vi "Add Device.vi"(8 "error in (no error)":errorcluster, 9 "J1939 Monitor Settings":T2 {"Name" format="%.0x"}, 10 "Name":string, 11 "NodeID":u64) -> (0 "error out":errorcluster, 2 "Device Ref out":T1 format="%.0x")   [LabVIEW 2023, in "J1939 System Definition API Support.lvlib"]
uses:
  J1939 System Definition API Support.lvlib
  Addon/Addon Shared/Types/Monitor Settings.ctl
  <vilib>/NI VeriStand/Custom Device API/Custom Device Item Ref.ctl
  Addon/Addon Shared/SubVIs/Constants.vi
  <vilib>/NI/NI VeriStand Advanced SysDef API/_SubVIs/SysDef.Search.GUID.vi
  Addon/Addon Shared/J1939 Addon Shared.lvlib
  <vilib>/NI/NI VeriStand Advanced SysDef API/SysDef API/Advanced System Definition.lvlib
  <vilib>/NI VeriStand/Custom Device API/Custom Device API.lvlib
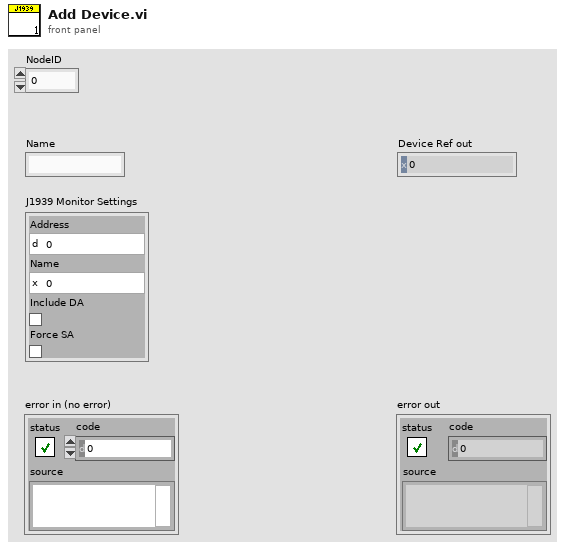
[diagram p1: front panel]
types:
  T1 = typedef "Custom Device API.lvlib/Custom Device Item Ref.ctl" = u64
  T2 = typedef "J1939 Addon Shared.lvlib/Monitor Settings.ctl" = cluster{"Address":u8, "Name":u64, "Include DA":bool, "Force SA":bool}
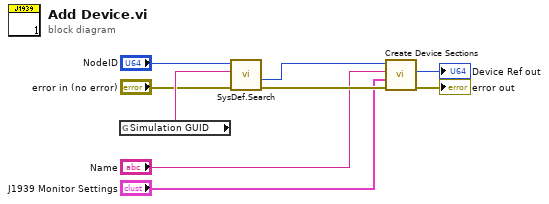
[diagram p0: block diagram]
diagram:
  n1 = global read "Constants.vi" "Simulation GUID"() -> (w9:string)
  n2 = call-poly <vilib>:"SysDef.Search.vi"("error in (no error)"="error in (no error)", "GUID"=w9, "nodeID"="NodeID") -> ("error out"=w8:errorcluster, "Value out"=w7:u64)  [unwired: 5 in, 2 out]
  n3 = call "Create Device Sections.vi"("error in (no error)"=w8, "J1939 Monitor Settings"="J1939 Monitor Settings", "Name"="Name", "Item Ref in"=w7) -> ("error out"=→"error out":errorcluster, "Device Ref out"=→"Device Ref out":T1)  [unwired: 6 in]
